vi "FPGA_ADC_config.vi"(1 "Inst_parameter":T2={"Kind"=0, "Strings"=["ADC", "", "V", "ADC0;ADC1", "V;V"], "uint64s"=[10, 2, 250000, 0, 100, 10106, 1000000], "Doubles"=[1.0], "DAQmx take out list"=[]}, 2 "FPGA ref in":T1) -> (0 "FPGA ref out":T1)   [LabVIEW 2013]
uses:
  fpga-bitfile-ref.ctl
  <vilib>/LabVIEW Targets/FPGA/cRIO/shared/nicrio_ModuleControls/nicrio_cRIO-9205_VoltageRange.ctl
  <vilib>/LabVIEW Targets/FPGA/cRIO/shared/nicrio_ModuleControls/nicrio_cRIO-9205_TerminalMode.ctl
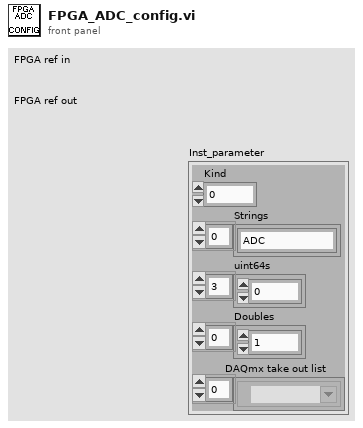
[diagram p1: front panel]
types:
  T1 = typedef "fpga-bitfile-ref.ctl" = refnum<k20>
  T2 = cluster{"Kind":u16, "Strings":string[], "uint64s":u64[], "Doubles":dbl[], "DAQmx take out list":refnum<k21>[]}
  T3 = cluster{"mode":enum8{"ramp", "RT"}, "source":u8, "edge":enum8{"falling", "rising", "both"}}
  T4 = typedef "nicrio_cRIO-9205_VoltageRange.ctl" = enum8{"+/- 10V", "+/- 5V", "+/- 1V", "+/- 200mV"}
  T5 = typedef "nicrio_cRIO-9205_TerminalMode.ctl" = enum8{"RSE", "NRSE", "DIFF"}
  T6 = cluster{"AI Channel":u8, "Voltage Range":T4, "Terminal Mode":T5}
  T7 = enum16{"empty", "stop", "start", "sampling rate", "trigger", "sample count", "reset channels", "add channel", "avg per point"}
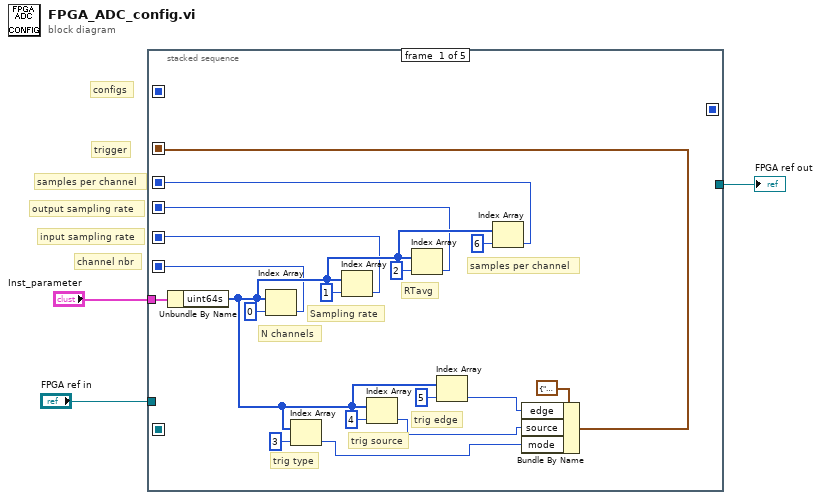
[diagram p0: block diagram]
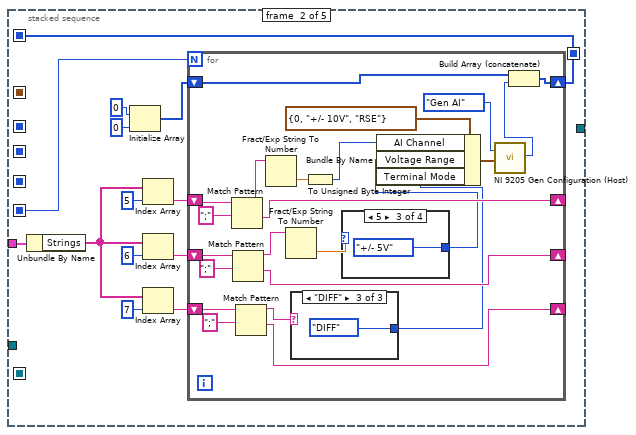
[diagram p2: hidden frame]
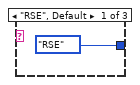
[diagram p3: hidden frame]
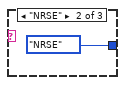
[diagram p4: hidden frame]
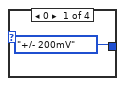
[diagram p5: hidden frame]
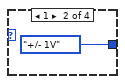
[diagram p6: hidden frame]
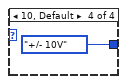
[diagram p7: hidden frame]
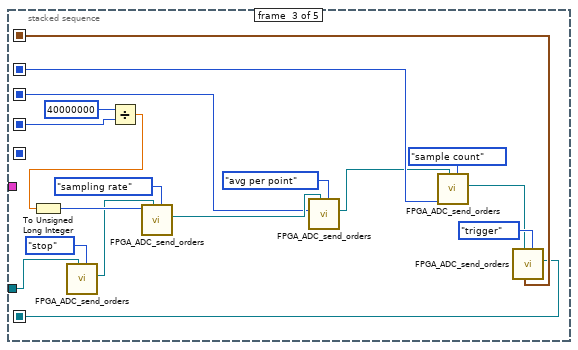
[diagram p8: hidden frame]
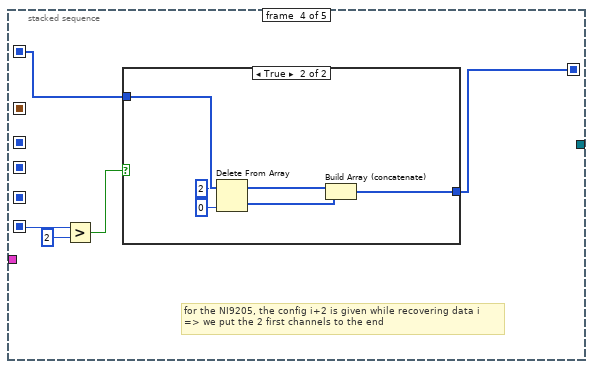
[diagram p9: hidden frame]
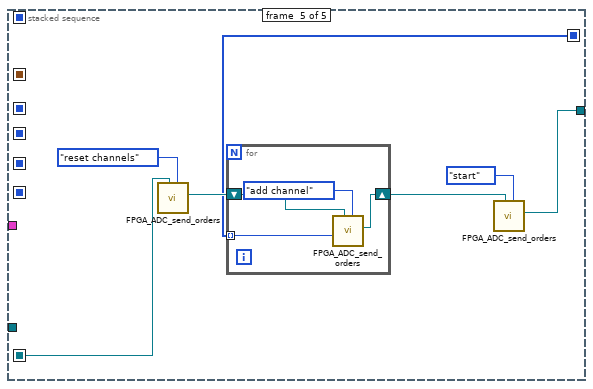
[diagram p11: hidden frame]
diagram:
  # "configs"
  # "trigger"
  # "samples per channel"
  # "output sampling rate"
  # "input sampling rate"
  # "channel nbr"
  n1 = stacked-sequence {
    seq-local: [w8 _ _ _ _] -> [_ w26 _ w87 _]
    seq-local: [w7 _ _ _ _] -> [_ _ w67 _ _]
    seq-local: [w5 _ _ _ _] -> [_ _ w66 _ _]
    seq-local: [w6 _ _ _ _] -> [_ _ w72 _ _]
    seq-local: [w4 _ _ _ _] -> [_ _ w75 _ _]
    seq-local: [_ w22 _ _ _] -> [_ _ _ w84 _]
    seq-local: [_ _ w74 _ _] -> [_ _ _ _ w99]
    seq-local: [_ _ _ w83 _] -> [_ _ _ _ w95]
    tunnel: "Inst_parameter" -> [w21 w34 _ _ _]
    tunnel: [_ _ _ _ w96] -> w1
    tunnel: "FPGA ref in" -> [_ _ w77 _ _]
    frame #0 {
      # "samples per channel"
      # "trig edge"
      # "trig source"
      # "trig type"
      # "RTavg"
      # "Sampling rate"
      # "N channels"
      n2 = Unbundle By Name(w21) -> ("uint64s"=w9:u64[])
      n3 = Index Array(array=w9, index=0) -> (element=w8:u64)
      n4 = Index Array(array=w9, index=3) -> (element=w13:u64)
      n5 = Index Array(array=w9, index=1) -> (element=w7:u64)
      n6 = Index Array(array=w9, index=4) -> (element=w11:u64)
      n7 = Index Array(array=w9, index=2) -> (element=w5:u64)
      n8 = Index Array(array=w9, index=5) -> (element=w12:u64)
      n9 = Index Array(array=w9, index=6) -> (element=w6:u64)
      n10 = Bundle By Name(cluster=T3 {"mode"=enum."ramp", "source"=1, "edge"=enum."falling"} ("Trigger 2"), "edge"=w12, "source"=w11, "mode"=w13) -> (w4:T3)
    }
    frame #1 {
      n11 = Unbundle By Name(w34) -> ("Strings"=w27:string[])
      n12 = Initialize Array(u16 0 ("IO Sample\nConfiguration"), 0 ("dimension size")) -> (w24:u16[])
      n13 = Index Array(array=w27, index=5) -> (element=w32:string)
      n14 = Index Array(array=w27, index=6) -> (element=w31:string)
      n15 = Index Array(array=w27, index=7) -> (element=w28:string)
      n16 = for {
        N: w26 -> [_]
        shift-right: [w55] -> _
        shift-left: w32 -> [w54]
        shift-right: [w44] -> _
        shift-left: w31 -> [w47]
        shift-right: [w39] -> _
        shift-left: w28 -> [w42]
        shift-right: [w37] -> w22
        shift-left: w24 -> [w36]
        n17 = Match Pattern(string=w54, regular expression=";") -> (before substring=w56:string, after substring=w55:string)  [unwired: 1 in, 2 out]
        n18 = Match Pattern(string=w47, regular expression=";") -> (before substring=w49:string, after substring=w44:string)  [unwired: 1 in, 2 out]
        n19 = Match Pattern(string=w42, regular expression=";") -> (before substring=w41:string, after substring=w39:string)  [unwired: 1 in, 2 out]
        n20 = Fract/Exp String To Number(string=w56) -> (number=w52:dbl)  [unwired: 3 in, 1 out]
        n21 = Fract/Exp String To Number(string=w49) -> (number=w46:dbl)  [unwired: 3 in, 1 out]
        n22 = case shown="\"DIFF\"" w41 {
          tunnel: [nicrio_cRIO-9205_TerminalMode."RSE" ("Terminal Mode") nicrio_cRIO-9205_TerminalMode."NRSE" ("Terminal Mode") nicrio_cRIO-9205_TerminalMode."DIFF" ("Terminal Mode")] -> w40
          frame "RSE", Default {
          }
          frame "NRSE" {
          }
          frame "DIFF" {
          }
        }
        n23 = To Unsigned Byte Integer(number=w52) -> (unsigned 8bit integer=w51:u8)
        n24 = case shown="5" w46 {
          tunnel: [nicrio_cRIO-9205_VoltageRange."+/- 200mV" ("Voltage Range") nicrio_cRIO-9205_VoltageRange."+/- 1V" ("Voltage Range") nicrio_cRIO-9205_VoltageRange."+/- 5V" ("Voltage Range") nicrio_cRIO-9205_VoltageRange."+/- 10V" ("Voltage Range")] -> w45
          frame 0 {
          }
          frame 1 {
          }
          frame 5 {
          }
          frame 10, Default {
          }
        }
        n25 = Bundle By Name(cluster=T6 {"AI Channel"=0, "Voltage Range"=enum."+/- 10V", "Terminal Mode"=enum."RSE"} ("AI Channel and Settings"), "AI Channel"=w51, "Voltage Range"=w45, "Terminal Mode"=w40) -> (w50:T6)
        n26 = call "NI 9205 Gen Configuration (Host).vi"("Gen Type"=enum8{"Gen AI", "Gen DI", "Gen DO"}."Gen AI", "AI Channel and Settings"=w50) -> ("IO Sample\nConfiguration"=w35:u16)  [unwired: 17 in]
        n27 = Build Array (concatenate)(w36, w35) -> (w37:u16[])
      }
    }
    frame #2 {
      n28 = call "FPGA_ADC_send_orders.vi"("option"=T7."stop", "FPGA VI Reference In"=w77) -> ("FPGA VI Reference Out"=w78:T1)  [unwired: 8 in, 1 out]
      n29 = Divide(x=u64 40000000, y=w67) -> (x/y=w65:dbl)
      n30 = To Unsigned Long Integer(number=w65) -> (unsigned 32bit integer=w79:u32)
      n31 = call "FPGA_ADC_send_orders.vi"("option"=T7."sampling rate", "FPGA VI Reference In"=w78, "40MHz divider"=w79) -> ("FPGA VI Reference Out"=w69:T1)  [unwired: 7 in, 1 out]
      n32 = call "FPGA_ADC_send_orders.vi"("option"=T7."avg per point", "FPGA VI Reference In"=w69, "avg per point"=w66) -> ("FPGA VI Reference Out"=w68:T1)  [unwired: 7 in, 1 out]
      n33 = call "FPGA_ADC_send_orders.vi"("option"=T7."sample count", "FPGA VI Reference In"=w68, "sample count"=w72) -> ("FPGA VI Reference Out"=w71:T1)  [unwired: 7 in, 1 out]
      n34 = call "FPGA_ADC_send_orders.vi"("option"=T7."trigger", "Trigger"=w75, "FPGA VI Reference In"=w71) -> ("FPGA VI Reference Out"=w74:T1)  [unwired: 7 in, 1 out]
    }
    frame #3 {
      # "for the NI9205, the config i+2 is given while recovering data i\n=> we put the 2 first channels to the end"
      n35 = Greater?(x=w87, y=u64 2) -> (0:w86:bool)
      n36 = case shown="True" w86 {
        tunnel: w84 -> [w88 w94]
        tunnel: [w88 w89] -> w83
        frame False {
        }
        frame True {
          n37 = Delete From Array(array=w94, length=2, index=0) -> (deleted portion=w90:u16[], array with subset deleted=w91:u16[])
          n38 = Build Array (concatenate)(w91, w90) -> (w89:u16[])
        }
      }
    }
    frame #4 {
      n39 = call "FPGA_ADC_send_orders.vi"("option"=T7."reset channels", "FPGA VI Reference In"=w99) -> ("FPGA VI Reference Out"=w100:T1)  [unwired: 8 in, 1 out]
      n40 = for {
        tunnel: w95 -> [w104] mode=indexing
        shift-right: [w103] -> w97
        shift-left: w100 -> [w102]
        n41 = call "FPGA_ADC_send_orders.vi"("option"=T7."add channel", "FPGA VI Reference In"=w102, "channel config"=w104) -> ("FPGA VI Reference Out"=w103:T1)  [unwired: 7 in, 1 out]
      }
      n42 = call "FPGA_ADC_send_orders.vi"("option"=T7."start", "FPGA VI Reference In"=w97) -> ("FPGA VI Reference Out"=w96:T1)  [unwired: 8 in, 1 out]
    }
  }
  "FPGA ref out" <- w1
